vi "Coord window-Offsets entry window.vi"() -> (0 "Cancelled":bool, 1 "Z offset out":dbl, 2 "Y offset out":dbl, 3 "X offset out":dbl)   [LabVIEW 2020]
doc: "Use this template to create a dialog box with event handling."
uses:
  <vilib>/Utility/miscctls.llb/LVPointTypeDef.ctl
  Global Variables/General Globals.vi
panel:
  in  "Z offset":dbl
  in  "Y offset":dbl
  in  "Cancel":bool
  in  "OK":bool
  in  "X offset":dbl
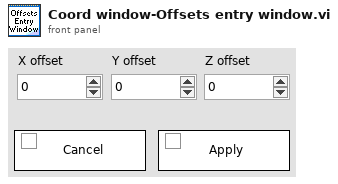
[diagram p1: front panel]
types:
  T1 = typedef "LVPointTypeDef.ctl" = cluster{"Horizontal":i16, "Vertical":i16}
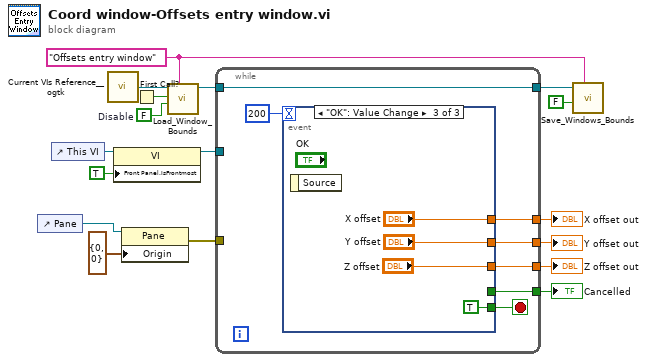
[diagram p0: block diagram]
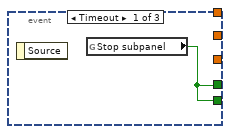
[diagram p2: hidden frame]
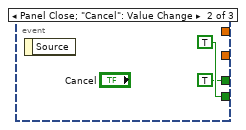
[diagram p3: hidden frame]
diagram:
  w8 = FALSE  # Disable
  w7 = "Offsets entry window" ("Window Name (i.e. Key)")
  n1 = control-ref of="Pane"() -> (w12:refnum<vi>)
  n2 = control-ref of="This VI"() -> (w16:refnum<vi>)
  n3 = call <userlib>:"Current VIs Reference__ogtk.vi"() -> ("Current VI's reference"=w10:refnum<vi>)  [unwired: 5 in]
  n4 = property on="Property Node" class="VI"(reference=w16, "Front Panel.IsFrontmost"=TRUE ("Front Panel Window:Is Frontmost")) -> (reference out=w15:refnum<vi>)  [unwired: 1 in, 1 out]
  n5 = property on="Property Node" class="Pane"(reference=w12, "Origin"=T1 {"Horizontal"=0, "Vertical"=0}) -> (error out=w13:errorcluster)  [unwired: 1 in, 1 out]
  n6 = First Call?() -> (First Call?: T/F=w9:bool)
  n7 = call "Load_Window_Bounds.vi"("Window Name (i.e. Key)"=w7, "Disable"=w8, "First Call"=w9, "Window VI's Ref"=w10) -> ("reference out"=w5:refnum<vi>)  [unwired: 4 in, 3 out]
  n8 = while {
    tunnel: w13 -> [_]
    tunnel: w15 -> [_]
    tunnel: [w22] -> w11
    tunnel: w5 -> [w21]
    tunnel: [w21] -> w4
    tunnel: [w20] -> w3
    tunnel: [w19] -> w2
    tunnel: [w18] -> w1
    stop <- w24 stop-if-true
    n9 = event shown="[2] \"OK\": Value Change" {
      selector: _ -> [_ _ _]
      dyn-events: _ -> [_ _ _]
      timeout: 200 -> [_ _ _]
      tunnel: [w25 TRUE ("Stop?") TRUE ("Stop?")] -> w24
      tunnel: [w25 TRUE ("Stop subpanel") _] -> w22
      tunnel: [_ _ "X offset"] -> w20
      tunnel: [_ _ "Y offset"] -> w19
      tunnel: [_ _ "Z offset"] -> w18
      event Timeout {
        n10 = event-data() -> ()  [unwired: 1 in, 1 out]
        n11 = global read "General Globals.vi" "Stop subpanel"() -> (w25:bool)
      }
      event Panel Close; "Cancel": Value Change {
        n12 = event-data() -> ()  [unwired: 1 in, 1 out]
      }
      event "OK": Value Change {
        n13 = event-data() -> ()  [unwired: 1 in, 1 out]
      }
    }
  }
  "Cancelled" <- w11
  "X offset out" <- w3
  "Y offset out" <- w2
  "Z offset out" <- w1
  n14 = call "Save_Windows_Bounds.vi"("Window Name (i.e. Key)"=w7, "Front Panel Window:Open"=FALSE, "Window VI's Ref"=w4) -> ()  [unwired: 8 in, 1 out]
